vi "ATC_SEL.vi"(8 "error in":errorcluster, 11 "ATC_0/1_OFF/ON":u16(ring)=1 items=["Enable"=1, "Disable"=0]) -> (0 "error out":errorcluster)   [LabVIEW 2023]
panel:
  in  "TCPIPin":T1={"address"="192.168.100.111", "remote port or service name"=5025, "timeout ms (60000)"=10000}
  # "CLC_Gen4_L2"
  # "/* SCPI command: ATC_SEL\n        * Parameters:\n        *  param: 0 to disable, 1 to enable\n        *\n        * Example usage:\n        * ATC_SEL 0  // Disable ATC\n        * ATC_SEL 1  // Enable ATC\n        */"
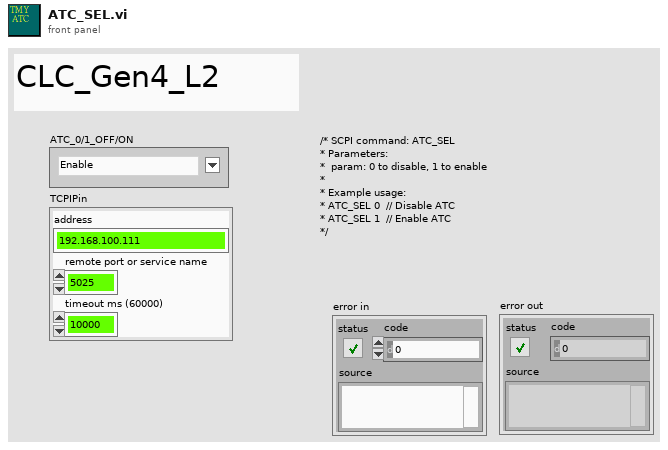
[diagram p1: front panel]
types:
  T1 = cluster{"address":string, "remote port or service name":u16, "timeout ms (60000)":i32}
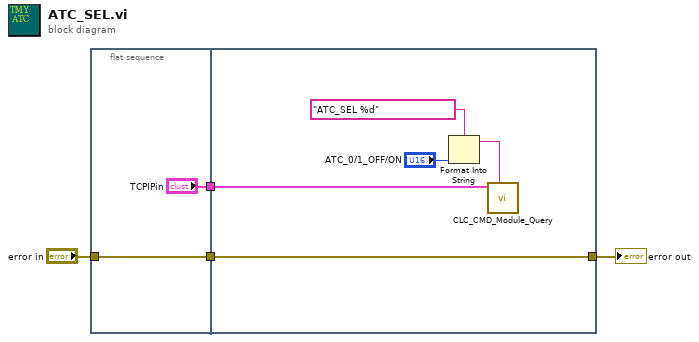
[diagram p0: block diagram]
diagram:
  n1 = flat-sequence {
    tunnel: ["TCPIPin"] -> w4
    tunnel: "error in" -> [w5]
    tunnel: [w5] -> w2
    tunnel: w2 -> [w7]
    tunnel: w4 -> [w8]
    tunnel: [w7] -> w1
    frame #0 {
    }
    frame #1 {
      n2 = Format Into String(format string="ATC_SEL %d" ("data in"), "ATC_0/1_OFF/ON") -> (resulting string=w9:string)  [unwired: 2 in, 1 out]
      n3 = call "CLC_CMD_Module_Query.vi"("CMD in"=w9, "TCPIPin"=w8) -> ()  [unwired: 7 in, 3 out]
    }
  }
  "error out" <- w1
